vi "Convert Norm FOV to FOV.vi"(11 "Field of View(norm)":dbl=4.35) -> (2 "FOV":dbl)   [LabVIEW 2017]
uses:
  Global Variables/General Globals.vi
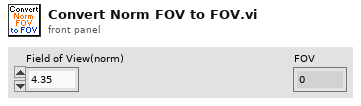
[diagram p1: front panel]
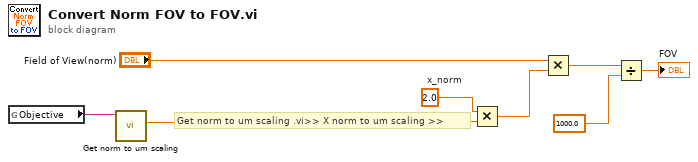
[diagram p0: block diagram]
diagram:
  w6 = 2.0  # x_norm
  # "Get norm to um scaling .vi>> X norm to um scaling >>"
  n1 = global read "General Globals.vi" "Objective"() -> (w5:string)
  n2 = call "Get norm to um scaling .vi"("Current Objective"=w5) -> ("X_norm to um_scaling"=w7:dbl)  [unwired: 8 in, 2 out]
  n3 = Multiply(x=w6, y=w7) -> (x*y=w4:dbl)
  n4 = Multiply(x="Field of View(norm)", y=w4) -> (x*y=w3:dbl)
  n5 = Divide(x=w3, y=1000.0) -> (x/y=→"FOV":dbl)
